vi "GUI DAQ Write.vi"(8 "error in (no error)":errorcluster, 10 "GUI Refs":T1, 11 "View Model":T2) -> (0 "error out":errorcluster, 3 "View Model":T2)   [LabVIEW 2017]
doc: "Store DAQ data from GUI arrays of clusters into DVR"
uses:
  View Model/Controls/View Model.ctl
  View Model/Controls/Shared Model.ctl
  Error Handler/Controls/Error Model.ctl
  Error Handler/Controls/Error Event.ctl
  Error Handler/Controls/Error Type.ctl
  Controller/Controls/Controller Model.ctl
  Controller/Controls/Controller Event.ctl
  Controller/Controls/Controller Command.ctl
  Controller/Controls/Controller Overhead.ctl
  Real-Time/RT Status.ctl
  Real-Time/RT Loop Status.ctl
  Controller/Controls/Controller NStream.ctl
  Controller/Controls/Controller DAQ Data.ctl
  TDMS Logger/Controls/TDMS Model.ctl
  TDMS Logger/Controls/TDMS Event.ctl
  TDMS Logger/Controls/TDMS Command.ctl
  TDMS Logger/Controls/TDMS Overhead.ctl
  TDMS Logger/Controls/TDMS ChanProperties.ctl
  Controls/GUI Referencies.ctl
  Controls/Discrete_GUI_Cluster.ctl
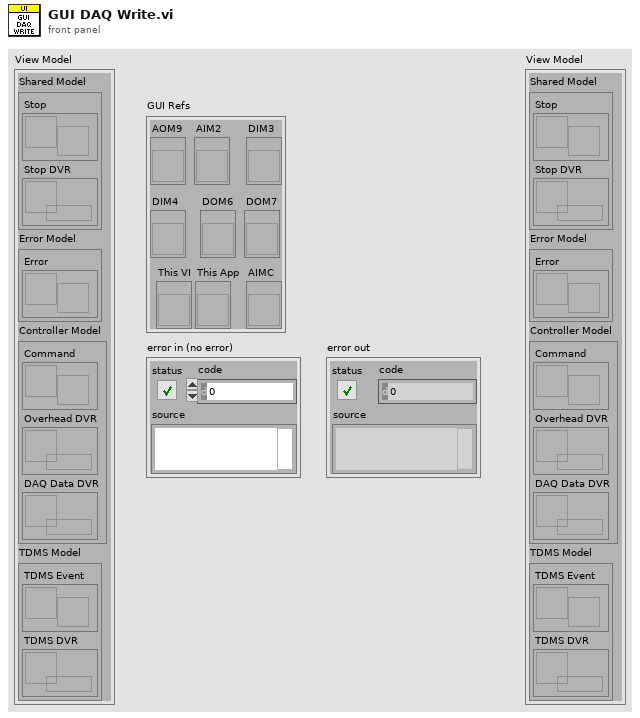
[diagram p1: front panel]
types:
  T1 = typedef "GUI Referencies.ctl" = cluster{"This VI":refnum<vi>, "This App":refnum<vi>, "DIM3":refnum<vi>, "DIM4":refnum<vi>, "DOM6":refnum<vi>, "DOM7":refnum<vi>, "AOM9":refnum<vi>, "AIM2":refnum<vi>, "AIMC":refnum<vi>}
  T2 = typedef "View Model.ctl" = cluster{"Shared Model":T3, "Error Model":T4, "Controller Model":T5, "TDMS Model":T6}
  T3 = typedef "Shared Model.ctl" = cluster{"Stop":refnum<user-event>, "Stop DVR":refnum<data-value>}
  T4 = typedef "Error Model.ctl" = cluster{"Error":refnum<user-event>}
  T5 = typedef "Controller Model.ctl" = cluster{"Command":refnum<user-event>, "Overhead DVR":refnum<data-value>, "DAQ Data DVR":refnum<data-value>}
  T6 = typedef "TDMS Model.ctl" = cluster{"TDMS Event":refnum<user-event>, "TDMS DVR":refnum<data-value>}
  T7 = typedef "Discrete_GUI_Cluster.ctl" = cluster{"Ch.name":string, "Ch.state":bool, "Num":string}
  T8 = typedef "AIMV_GUI_Cluster.ctl" = cluster{"Ch.name":string, "Ch.value":dbl, "Ch.range":string, "Num":string}
  T9 = typedef "AIMC_GUI_Cluster.ctl" = cluster{"Ch.name":string, "Ch.value":dbl, "Ch.range":string, "Num":string}
  T10 = typedef "Controller DAQ Data.ctl" = cluster{"AOM data":dbl[], "AIMV data":dbl[], "AIMC data":dbl[], "DOM data":dbl[], "DIM data":dbl[], "AOM timestamp":dbl, "AIMV timestamp":dbl, "AIMC timestamp":dbl, "DOM timestamp":dbl, "DIM timestamp":dbl}
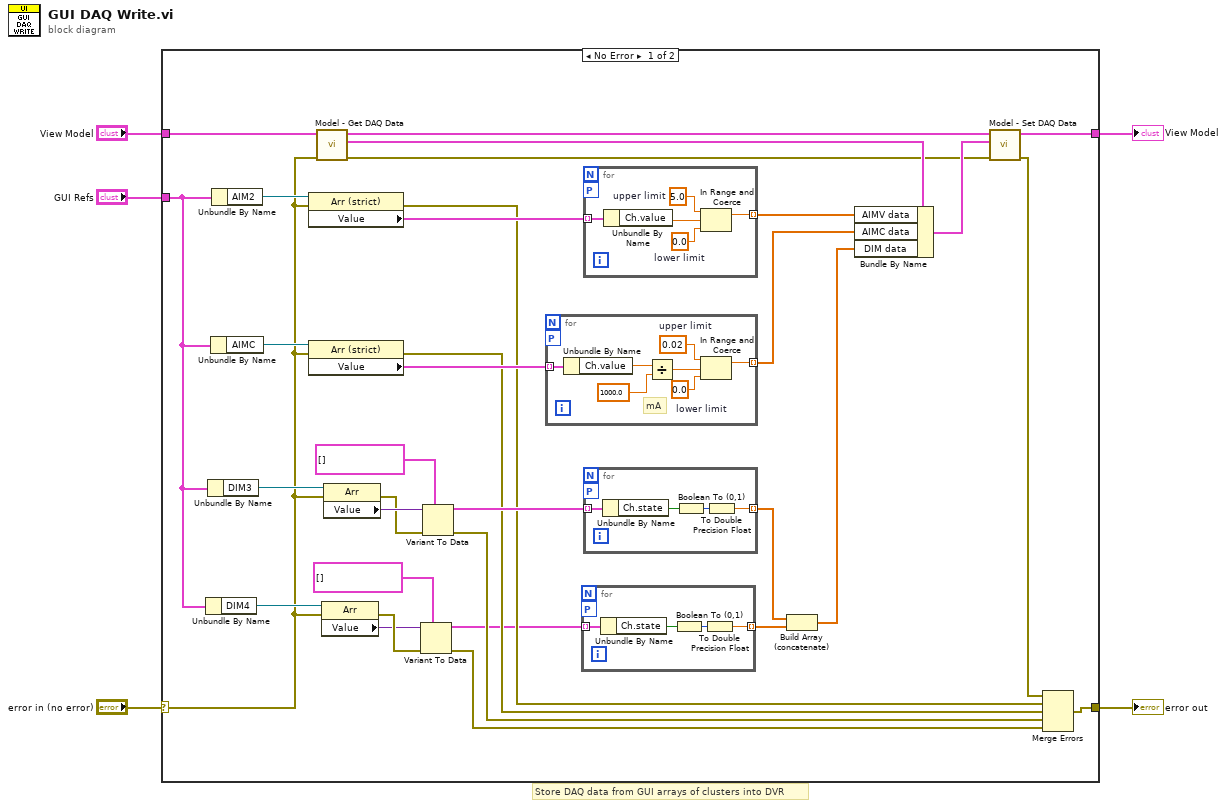
[diagram p0: block diagram]
diagram:
  # "Store DAQ data from GUI arrays of clusters into DVR"
  n1 = case shown="No Error" "error in (no error)" {
    selector: "error in (no error)" -> [w11 w59]
    tunnel: [w18 w59] -> w4
    tunnel: "View Model" -> [w22 w60]
    tunnel: [w26 w60] -> w2
    tunnel: "GUI Refs" -> [w10 _]
    frame No Error {
      n2 = Unbundle By Name(w10) -> ("DIM4"=w12:refnum<vi>)
      n3 = Unbundle By Name(w10) -> ("DIM3"=w34:refnum<vi>)
      n4 = Unbundle By Name(w10) -> ("AIMC"=w35:refnum<vi>)
      n5 = Unbundle By Name(w10) -> ("AIM2"=w38:refnum<vi>)
      n6 = property class="Arr (strict)"(reference=w38, error in=w11) -> (error out=w23:errorcluster, "Value"=w37:T8[])  [unwired: 1 out]
      n7 = property class="Arr (strict)"(reference=w35, error in=w11) -> (error out=w24:errorcluster, "Value"=w36:T9[])  [unwired: 1 out]
      n8 = call "Model - Get DAQ Data.vi"("error in (no error)"=w11, "View Model"=w22) -> ("error out"=w19:errorcluster, "DAQ Data"=w20:T10, "View Model"=w21:T2)  [unwired: 7 in]
      n9 = property class="Arr"(reference=w12, error in=w11) -> (error out=w14:errorcluster, "Value"=w13:variant)  [unwired: 1 out]
      n10 = property class="Arr"(reference=w34, error in=w11) -> (error out=w32:errorcluster, "Value"=w33:variant)  [unwired: 1 out]
      n11 = Variant To Data(error in=w14, type=T7[] [], Variant=w13) -> (data=w16:T7[], error out=w9:errorcluster)
      n12 = Variant To Data(error in=w32, type=T7[] [], Variant=w33) -> (data=w30:T7[], error out=w25:errorcluster)
      n13 = for {
        tunnel: w36 -> [w53] mode=indexing
        tunnel: [w50] -> w28 mode=indexing
        workers-P: _ -> [_]
        w51 = 0.0  # lower limit
        w52 = 0.02  # upper limit
        # "mA"
        n14 = Unbundle By Name(w53) -> ("Ch.value"=w49:dbl)
        n15 = Divide(x=w49, y=1000.0) -> (x/y=w47:dbl)
        n16 = In Range and Coerce(upper limit=w52, x=w47, lower limit=w51) -> (coerced(x)=w50:dbl)  [unwired: 1 out]
      }
      n17 = for {
        tunnel: w16 -> [w42] mode=indexing
        tunnel: [w39] -> w8 mode=indexing
        workers-P: _ -> [_]
        n18 = Unbundle By Name(w42) -> ("Ch.state"=w40:bool)
        n19 = Boolean To (0,1)(Boolean=w40) -> (0, 1=w41:i16)
        n20 = To Double Precision Float(number=w41) -> (double precision float=w39:dbl)
      }
      n21 = for {
        tunnel: w37 -> [w58] mode=indexing
        tunnel: [w54] -> w29 mode=indexing
        workers-P: _ -> [_]
        w55 = 0.0  # lower limit
        w56 = 5.0  # upper limit
        n22 = Unbundle By Name(w58) -> ("Ch.value"=w57:dbl)
        n23 = In Range and Coerce(upper limit=w56, x=w57, lower limit=w55) -> (coerced(x)=w54:dbl)  [unwired: 1 out]
      }
      n24 = for {
        tunnel: w30 -> [w46] mode=indexing
        tunnel: [w43] -> w7 mode=indexing
        workers-P: _ -> [_]
        n25 = Unbundle By Name(w46) -> ("Ch.state"=w44:bool)
        n26 = Boolean To (0,1)(Boolean=w44) -> (0, 1=w45:i16)
        n27 = To Double Precision Float(number=w45) -> (double precision float=w43:dbl)
      }
      n28 = Build Array (concatenate)(w7, w8) -> (w6:dbl[])
      n29 = Bundle By Name(cluster=w20, "AIMV data"=w29, "AIMC data"=w28, "DIM data"=w6) -> (w27:T10)
      n30 = call "Model - Set DAQ Data.vi"("error in (no error)"=w19, "DAQ Data"=w27, "View Model"=w21) -> ("error out"=w17:errorcluster, "View Model"=w26:T2)  [unwired: 7 in]
      n31 = Merge Errors(w17, w23, w24, w25, w9) -> (w18:errorcluster)
    }
    frame Error {
    }
  }
  "View Model" <- w2
  "error out" <- w4
